vi "Signaling RMS.vi"(0 "phase voltage spectra":T2(array[cluster]), 5 "signaling frequency (216.66 Hz)":dbl=216.66, 9 "system info in":refnum<class "EP System Info.lvclass">, 11 "error in (no error)":errorcluster) -> (4 "signaling voltage RMS values":dbl[](array[numeric]), 10 "system info out":refnum<class "EP System Info.lvclass">, 15 "error out":errorcluster)   [LabVIEW 2014, in "NI_EP_Power Quality.lvlib"]
doc: "Calculates the RMS voltage at a specified frequency of a complex voltage spectrum, according to IEC 61000-4-30:2008. The specified frequency corresponds to the signaling voltage.\n\nThis VI supports measuring single-line and multiple-line systems."
uses:
  <vilib>/addons/Electrical Power/PQ/NI_EP_Power Quality.lvlib
  <vilib>/addons/Electrical Power/PQ/Common/Controls/ep_AI Data Channel.ctl
  <vilib>/addons/Electrical Power/PQ/Common/Classes/System Info/EP System Info.lvclass
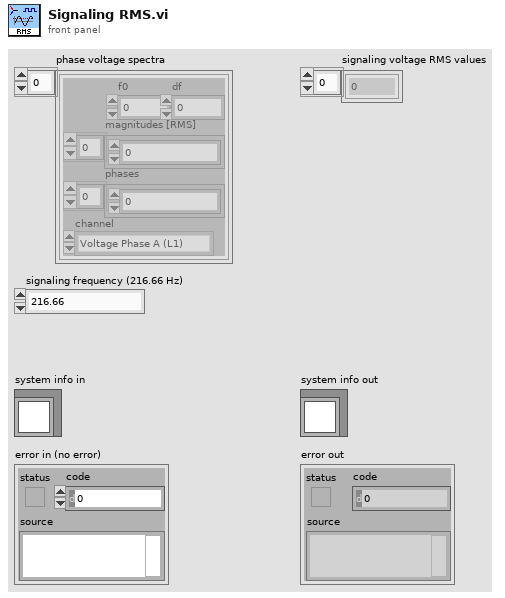
[diagram p1: front panel]
types:
  T1 = typedef "NI_EP_Power Quality.lvlib/ep_AI Data Channel.ctl" = enum16{"Voltage Phase A (L1)", "Voltage Phase B (L2)", "Voltage Phase C (L3)", "Voltage Phase N (Neutral)", "Current Phase A (L1)", "Current Phase B (L2)", "Current Phase C (L3)", "Current Phase N (Neutral)"}
  T2 = cluster{"f0":dbl, "df":dbl, "magnitudes [RMS]":dbl[], "phases":dbl[], "channel":T1}[]
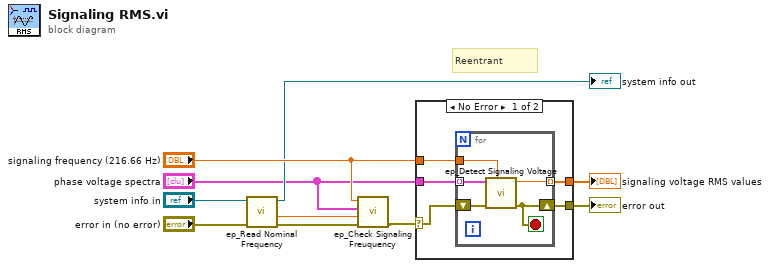
[diagram p0: block diagram]
diagram:
  # "Reentrant"
  n1 = call <vilib>:"ep_Read Nominal Frequency.vi"("error in (no error)"="error in (no error)", "system info in"="system info in") -> ("error out"=w2:errorcluster, "nominal frequency value"=w10:dbl, "system info out"=→"system info out":refnum<class "EP System Info.lvclass">)  [unwired: 6 in, 1 out]
  n2 = call <vilib>:"ep_Check Signaling Freuquency.vi"("error in (no error)"=w2, "nominal frequency value"=w10, "phase voltage spectra"="phase voltage spectra", "signaling frequency [Hz]"="signaling frequency (216.66 Hz)") -> ("error out"=w1:errorcluster)  [unwired: 7 in]
  n3 = case shown="No Error" w1 {
    selector: w1 -> [w12 w21]
    tunnel: "phase voltage spectra" -> [w15 _]
    tunnel: "signaling frequency (216.66 Hz)" -> [w14 _]
    tunnel: [w13 _] -> w8
    tunnel: [w11 w21] -> w7
    frame No Error {
      n4 = for {
        tunnel: w15 -> [w19] mode=indexing
        tunnel: w14 -> [w20]
        tunnel: [w18] -> w13 mode=indexing
        shift-right: [w16] -> w11
        shift-left: w12 -> [w17]
        stop <- w16 stop-if-true
        n5 = call <vilib>:"ep_Detect Signaling Voltage.vi"("signaling frequency"=w20, "error in (no error)"=w17, "voltage spectrum (5Hz step)"=w19) -> ("error out"=w16:errorcluster, "signaling voltage RMS [V]"=w18:dbl)  [unwired: 5 in, 2 out]
      }
    }
    frame Error {
    }
  }
  "error out" <- w7
  "signaling voltage RMS values" <- w8
